vi "Get or Add DefinedNames.vi"(8 "error in":errorcluster, 11 "SpreadsheetDoc in":refnum<k24>) -> (0 "error out":errorcluster, 2 "DefinedNames":refnum<k24>, 3 "SpreadsheetDoc out":refnum<k24>)   [LabVIEW 2021, in "Open Xml.lvlib"]
uses:
  Open Xml.lvlib
  D:/git/Open-Xml-LabVIEW/dll/DocumentFormat.OpenXml.dll
  dll/DocumentFormat.OpenXml.dll
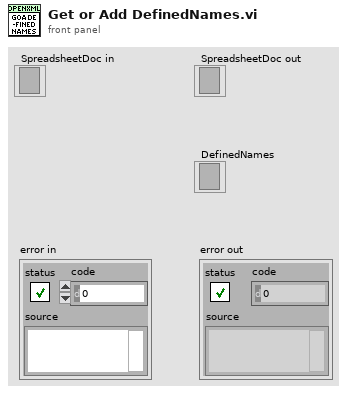
[diagram p1: front panel]
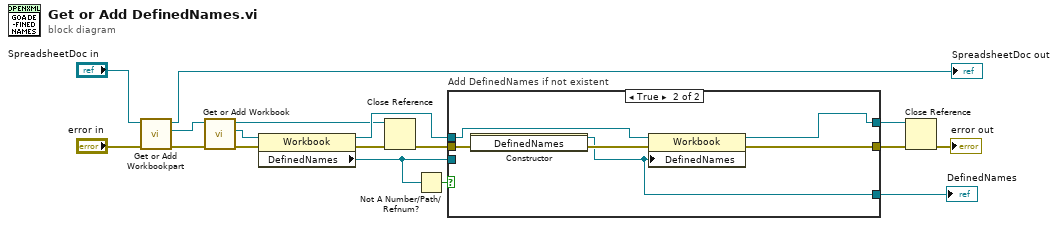
[diagram p0: block diagram]
diagram:
  n1 = call "Get or Add Workbookpart.vi"("error in"="error in", "SpreadsheetDoc in"="SpreadsheetDoc in") -> ("error out"=w9:errorcluster, "WorkbookPart"=w7:refnum<k24>, "SpreadsheetDoc out"=→"SpreadsheetDoc out":refnum<k24>)  [unwired: 7 in]
  n2 = call "Get or Add Workbook.vi"("error in"=w9, "Workbookpart in"=w7) -> ("error out"=w10:errorcluster, "Workbook"=w5:refnum<k24>, "Workbookpart out"=w3:refnum<k24>)  [unwired: 7 in]
  n3 = property class="Workbook"(reference=w5, error in=w10) -> (reference out=w12:refnum<k24>, error out=w11:errorcluster, "DefinedNames"=w13:refnum<k24>)
  n4 = Close Reference(reference=w3, error in (no error)=w11) -> (error out=w4:errorcluster)
  n5 = Not A Number/Path/Refnum?(number/path/refnum=w13) -> (NaN/Path/Refnum?=w14:bool)
  n6 = case "Add DefinedNames if not existent" shown="True" w14 {
    tunnel: w13 -> [w19 _]
    tunnel: w12 -> [w18 w26]
    tunnel: w4 -> [w20 w25]
    tunnel: [w20 w22] -> w16
    tunnel: [w19 w23] -> w15
    tunnel: [w18 w21] -> w1
    frame False {
    }
    frame True {
      n7 = constructor class="DefinedNames"(error in=w25) -> (reference out=w23:refnum<k24>, error out=w24:errorcluster)  [unwired: 2 in, 1 out]
      n8 = property class="Workbook"(reference=w26, error in=w24, "DefinedNames"=w23) -> (reference out=w21:refnum<k24>, error out=w22:errorcluster)
    }
  }
  "DefinedNames" <- w15
  n9 = Close Reference(reference=w1, error in (no error)=w16) -> (error out=→"error out":errorcluster)
